vi "Geometric Inverse CDF.vi"(10 "p":dbl=0.5, 11 "cdf(n)":dbl=0.4) -> (0 "error":i32, 3 "n":i32)   [LabVIEW 2018, in "NI_Gmath.lvlib"]
doc: "Computes the discrete inverse cumulative distribution function (CDF), or the value <B>x</B> such that the probability that the random variate X, where X describes the selected distribution type, takes on a value less than or equal to it is <B>cdf(x)</B>. You must manually select the polymorphic instance to use."
uses:
  NI_Gmath.lvlib
panel:
  # "Geometric Inverse CDF"
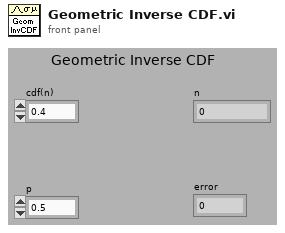
[diagram p1: front panel]
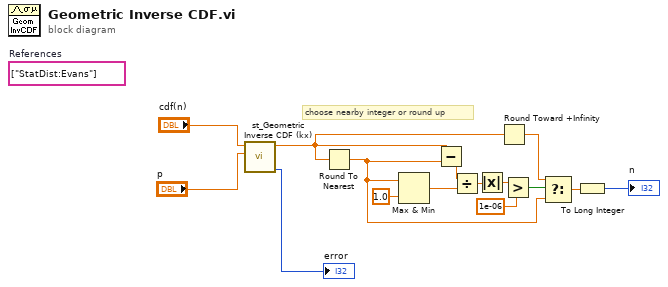
[diagram p0: block diagram]
diagram:
  (unwired) string[] ["StatDist:Evans"]  # References
  # "choose nearby integer or round up"
  n1 = call "st_Geometric Inverse CDF (kx).vi"("p"="p", "cdf(nx)"="cdf(n)") -> ("error"=→"error":i32, "nx"=w7:dbl)  [unwired: 8 in]
  n2 = Round To Nearest(number=w7) -> (nearest integer value=w3:dbl)
  n3 = Max & Min(x=w3, y=1.0) -> (max(x,y)=w1:dbl)  [unwired: 1 out]
  n4 = Subtract(x=w7, y=w3) -> (x-y=w13:dbl)
  n5 = Divide(x=w13, y=w1) -> (x/y=w11:dbl)
  n6 = Absolute Value(x=w11) -> (abs(x)=w12:dbl)
  n7 = Round Toward +Infinity(x=w7) -> (ceil(x): smallest int >= x=w8:dbl)
  n8 = Greater?(x=w12, y=1e-06) -> (0:w9:bool)
  n9 = Select(t=w8, s=w9, f=w3) -> (s? t:f=w14:dbl)
  n10 = To Long Integer(number=w14) -> (32bit integer=→"n":i32)
